vi "Open.vi"(8 "error in (no error)":errorcluster, 10 "address":string, 11 "Instrument.KH7008 in":refnum<class "Instrument.KH7008.lvclass">) -> (0 "error out":errorcluster, 3 "Instrument.KH7008 out":refnum<class "Instrument.KH7008.lvclass">)   [LabVIEW 2019, in "Instrument.KH7008.lvclass"]
uses:
  Instrument.KH7008.lvclass
  <userlib>/LevyLab/Instrument Framework/SMOs/Instrument/Instrument.lvclass
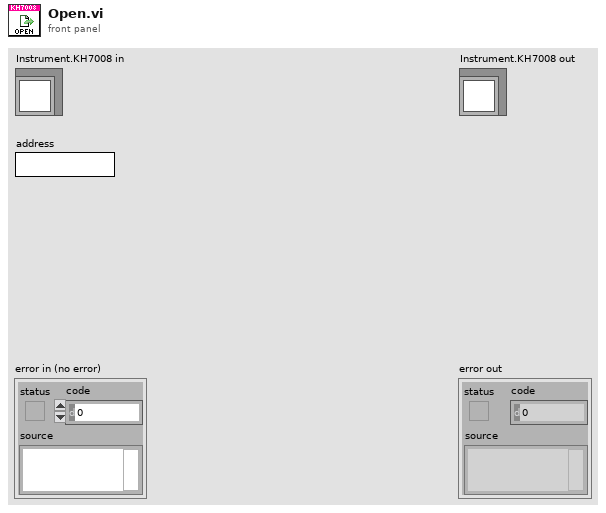
[diagram p1: front panel]
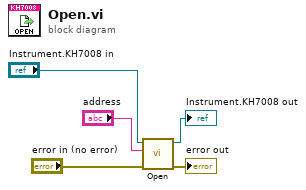
[diagram p0: block diagram]
diagram:
  n1 = call-parent "Open.vi"("error in (no error)"="error in (no error)", "address"="address", "Instrument in"="Instrument.KH7008 in") -> ("error out"=→"error out":errorcluster, "Instrument out"=→"Instrument.KH7008 out":refnum<class "Instrument.KH7008.lvclass">)  [unwired: 7 in]
